vi "Show Splash.vi"(8 "error in (no error)":errorcluster, 11 "Plugin Splash in":refnum<class "Plugin Splash.lvclass">) -> (0 "error out":errorcluster, 3 "Plugin Splash out":refnum<class "Plugin Splash.lvclass">)   [LabVIEW 2020, in "Volatus.lvlib" / "Plugin Splash.lvclass"]
uses:
  Plugin Splash.lvclass
  Plugin Splash.lvclass/Plugin Splash.ctl
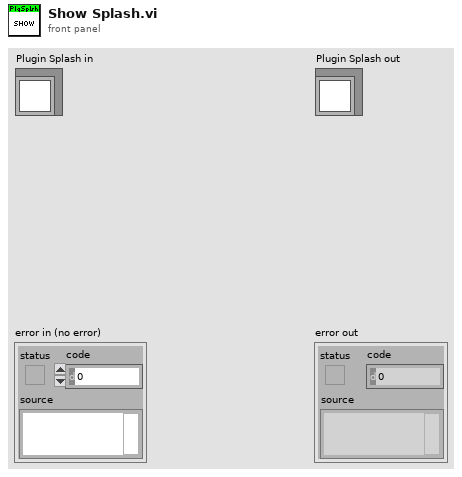
[diagram p1: front panel]
types:
  T1 = enum32{"Invalid", "Standard", "Closed", "Hidden", "Minimized", "Maximized"}
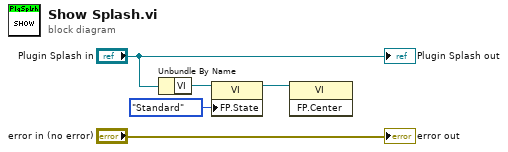
[diagram p0: block diagram]
diagram:
  n1 = Unbundle By Name("Plugin Splash in") -> ("VI"=w3:refnum<vi>)
  n2 = property class="VI"(reference=w3, "FP.State"=T1."Standard" ("Front Panel Window:State")) -> (reference out=w1:refnum<vi>)  [unwired: 1 in, 1 out]
  n3 = invoke class="VI" method="FP.Center"(reference=w1) -> ()  [unwired: 2 in, 3 out]
  "error out" <- "error in (no error)"
  "Plugin Splash out" <- "Plugin Splash in"
